vi "libssh2_channel_write_ex.vi"(8 "error in (no error)":errorcluster, 9 "buf":u8[](array[numeric]), 10 "stream_id":i32, 11 "channel":T1) -> (0 "error out":errorcluster, 3 "return value":i64)   [LabVIEW 2013, in "libssh2.lvlib"]
doc: "Writes data to a channel stream. All channel streams have one standard I/O substream (<B>stream_id</B> = 0), and may have up to 2^32 extended data streams as identified by the selected <B>stream_id</B>. The SSH2 protocol currently defines a stream ID of 1 to be the stderr substream."
uses:
  libssh2.lvlib
  Channel Refnum.ctl
  libssh2.dll
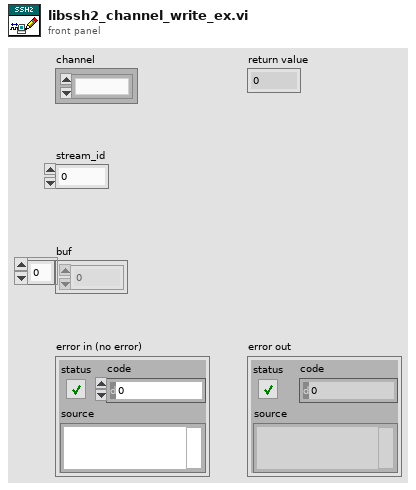
[diagram p1: front panel]
types:
  T1 = typedef "libssh2.lvlib/Channel Refnum.ctl" = refnum<k1>
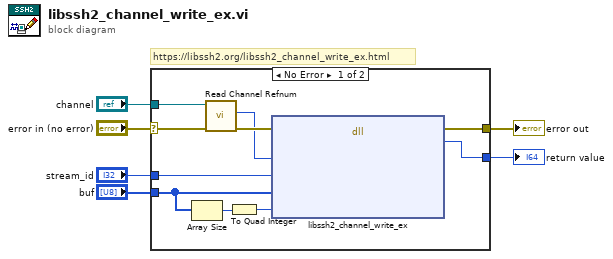
[diagram p0: block diagram]
diagram:
  # "https://libssh2.org/libssh2_channel_write_ex.html"
  n1 = case shown="No Error" "error in (no error)" {
    selector: "error in (no error)" -> [w7 w17]
    tunnel: [w16 w17] -> w6
    tunnel: "stream_id" -> [w15 _]
    tunnel: "buf" -> [w14 _]
    tunnel: [w12 _] -> w3
    tunnel: "channel" -> [w9 _]
    frame No Error {
      n2 = Array Size(array=w14) -> (size(s)=w13:i32)
      n3 = call "Read Channel Refnum.vi"("error in (no error)"=w7, "channel"=w9) -> ("error out"=w10:errorcluster, "LIBSSH2_CHANNEL*"=w8:u64)  [unwired: 8 in]
      n4 = To Quad Integer(1:w13) -> (0:w11:i64)
      n5 = dll-call lib="C:/Users/pasca/source/repos/libssh2-labview/libssh2**.*" fn="libssh2_channel_write_ex"(error in=w10, "channel"=w8, "stream_id"=w15, "buf"=w14, "buflen"=w11) -> (error out=w16:errorcluster, "return value"=w12:i64)  [unwired: 6 in, 1 out]
    }
    frame Error {
    }
  }
  "error out" <- w6
  "return value" <- w3
